vi "New.vi"(8 "error in (no error)":errorcluster, 11 "ModuleAdmin":refnum<class "ModuleAdmin.lvclass">) -> (0 "error out":errorcluster, 2 "First?":bool, 3 "ModuleAdmin":refnum<class "ModuleAdmin.lvclass">, 4 "Module ID":i32=-1)   [LabVIEW 2014, in "ModuleAdmin.lvlib" / "ModuleAdmin.lvclass"]
uses:
  ModuleAdmin.lvclass
  ModuleAdmin.lvclass/ModuleAdmin.ctl
  Accessors/Read CloneRegRef.vi
  Accessors/Write CloneRegRef.vi
  CloneRegistration/CloneRegistration.lvclass
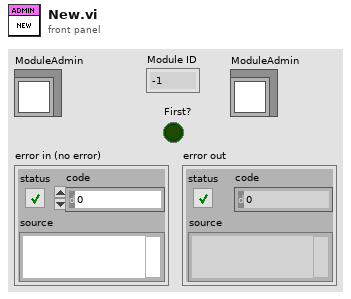
[diagram p1: front panel]
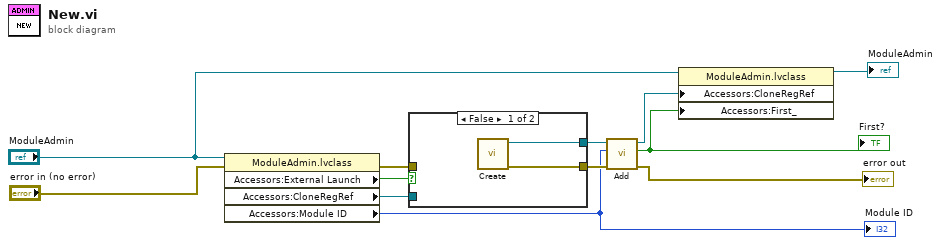
[diagram p0: block diagram]
diagram:
  n1 = property class="ModuleAdmin.lvclass"(reference="ModuleAdmin", error in="error in (no error)") -> (error out=w10:errorcluster, "Accessors:External Launch"=w11:bool, "Accessors:CloneRegRef"=w4:refnum<data-value>, "Accessors:Module ID"=w5:i32)  [unwired: 1 out]
  "Module ID" <- w5
  n2 = case shown="False" w11 {
    tunnel: w10 -> [_ w16]
    tunnel: [w14 w16] -> w9
    tunnel: w4 -> [_ w15]
    tunnel: [w13 w15] -> w3
    frame False {
      n3 = call "Create.vi"() -> ("error out"=w14:errorcluster, "CloneRegRef"=w13:refnum<data-value>)  [unwired: 10 in]
    }
    frame True {
      # "Init of Clone's registration\nhappened at Start Module.vi"
    }
  }
  n4 = call "Add.vi"("error in (no error)"=w9, "Module ID"=w5, "CloneRegRef"=w3) -> ("error out"=→"error out":errorcluster, "First?"=w1:bool, "CloneRegRef"=w2:refnum<data-value>)  [unwired: 6 in]
  "First?" <- w1
  n5 = property class="ModuleAdmin.lvclass"(reference="ModuleAdmin", "Accessors:CloneRegRef"=w2, "Accessors:First_"=w1) -> (reference out=→"ModuleAdmin":refnum<class "ModuleAdmin.lvclass">)  [unwired: 1 in, 1 out]
